vi "Quick Usb Set RS232Baud Rate.vi"(8 "error in (no error)":errorcluster, 10 "baudRate":u32, 11 "hDevice":u32) -> (0 "error out":errorcluster, 2 "function return":i32, 3 "hDevice out":u32)   [LabVIEW 2011, in "QuickUSB.lvlib"]
doc: "QUSBLIB QRETURN QuickUsbSetRS232BaudRate(\n QHANDLE hDevice, \n QULONG baudRate\n);"
uses:
  QuickUSB.lvlib
  QuickUSB.dll
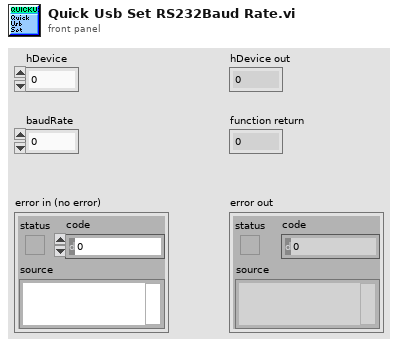
[diagram p1: front panel]
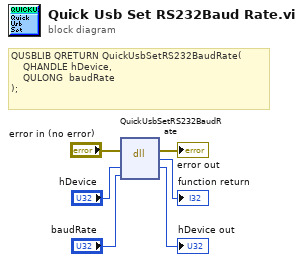
[diagram p0: block diagram]
diagram:
  # "QUSBLIB QRETURN QuickUsbSetRS232BaudRate(\n    QHANDLE hDevice, \n    QULONG  baudRate\n);"
  n1 = dll-call lib="C:/QuickUSB/QuickUSB.*" fn="QuickUsbSetRS232BaudRate"(error in="error in (no error)", "hDevice"="hDevice", "baudRate"="baudRate") -> (error out=→"error out":errorcluster, →"function return":i32, "hDevice"=→"hDevice out":u32)  [unwired: 3 in, 1 out]
